vi "Photo Calc Luminous Flux.vi"(7 "a_steradians":dbl, 8 "error in (no error)":errorcluster, 9 "a_distancecm":dbl, 10 "a_CIEResolution":u8, 11 "a_data":dbl[](array[numeric])) -> (0 "error out":errorcluster, 2 "function return":i16, 3 "a_data out":dbl[](array[numeric]), 4 "a_Lumen out":dbl)   [LabVIEW 2013, in "AVSirrad.lvlib"]
doc: "DLL_API short int __stdcall Photo_CalcLuminousFlux\n( \n DataType *a_data,\n unsigned char a_CIEResolution,\n double a_distancecm,\n double a_steradians,\n double *a_Lumen\n);"
uses:
  AVSirrad.lvlib
  AVSIRRAD/Examples/Labview/build/AVSirrad.dll
panel:
  in  "a_Lumen":dbl
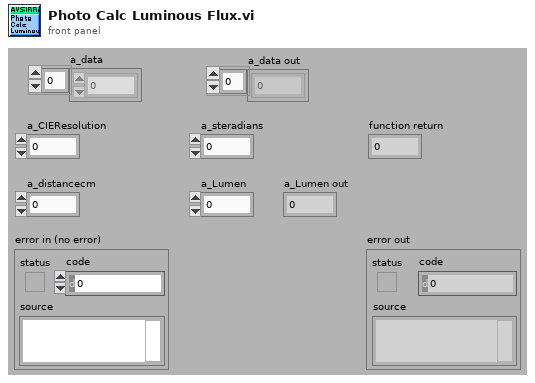
[diagram p1: front panel]
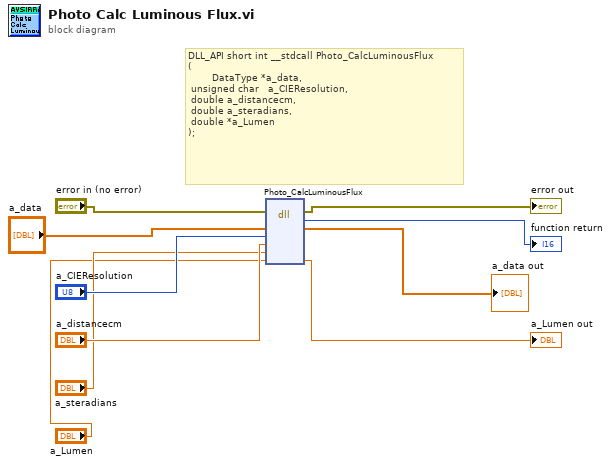
[diagram p0: block diagram]
diagram:
  # "DLL_API short int __stdcall Photo_CalcLuminousFlux\n( \n        DataType *a_data,\n\tunsigned char   a_CIEResolution,\n\tdouble a_distancecm,\n\tdouble a_steradians,\n\tdouble *a_Lumen\n);"
  n1 = dll-call lib="C:/AVSIRRAD/Examples/Labview/build/AVSirrad.*" fn="Photo_CalcLuminousFlux"(error in="error in (no error)", "a_data"="a_data", "a_CIEResolution"="a_CIEResolution", "a_distancecm"="a_distancecm", "a_steradians"="a_steradians", "a_Lumen"="a_Lumen") -> (error out=→"error out":errorcluster, "return type"=→"function return":i16, "a_data"=→"a_data out":dbl[], "a_Lumen"=→"a_Lumen out":dbl)  [unwired: 5 in, 1 out]
